vi "Center Insertion and IFFT.vi"(2 "Samples/Symbol":i32, 3 "Y(f) in":cdb[](array[numeric])) -> (0 "Freq Plot":dbl[](graph), 1 "Y(t) out":cdb[](array[numeric]))   [LabVIEW 2018]
uses:
  <vilib>/Analysis/NI_AALPro.lvlib
  <vilib>/Analysis/2dsp.llb/Inverse Complex FFT.vi
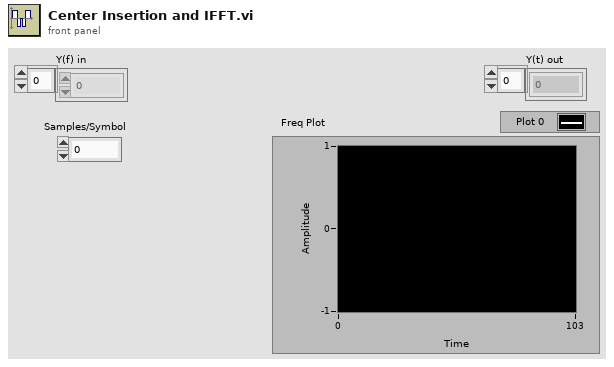
[diagram p1: front panel]
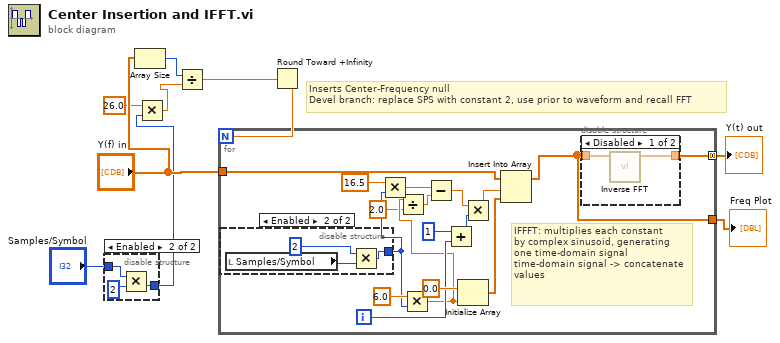
[diagram p0: block diagram]
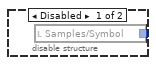
[diagram p3: hidden frame]
diagram:
  # "Inserts Center-Frequency null\nDevel branch: replace SPS with constant 2, use prior to waveform and recall FFT"
  n1 = disable-structure shown="Enabled" {
    disable-tunnel: [_ w13] -> w2
    disable-tunnel: "Samples/Symbol" -> [_ w11]
    frame Disabled {
    }
    frame Enabled {
      n2 = Multiply(x=w11, y=2) -> (x*y=w13:i32)
    }
  }
  n3 = Array Size(array="Y(f) in") -> (size(s)=w9:i32)
  n4 = Multiply(x=26.0, y=w2) -> (x*y=w3:dbl)
  n5 = Divide(x=w9, y=w3) -> (x/y=w10:dbl)
  n6 = Round Toward +Infinity(x=w10) -> (ceil(x): smallest int >= x=w8:dbl)
  n7 = for {
    N: w8 -> [_]
    tunnel: "Y(f) in" -> [w21]
    tunnel: [w23] -> w6 mode=concatenating
    tunnel: [w22] -> w5
    i -> [w27]
    # "IFFFT: multiplies each constant  \nby complex sinusoid, generating\none time-domain signal\ntime-domain signal -> concatenate values"
    n8 = disable-structure shown="Enabled" {
      disable-tunnel: [w31 w34] -> w19
      frame Disabled {
        n9 = local read "Samples/Symbol"() -> (w31:i32)
      }
      frame Enabled {
        n10 = local read "Samples/Symbol"() -> (w32:i32)
        n11 = Multiply(x=2 ("Samples/Symbol"), y=w32) -> (x*y=w34:i32)
      }
    }
    n12 = Multiply(x=16.5, y=w19) -> (x*y=w18:dbl)
    n13 = Multiply(x=6.0, y=w19) -> (x*y=w15:dbl)
    n14 = Divide(x=w15, y=2.0) -> (x/y=w16:dbl)
    n15 = Subtract(x=w18, y=w16) -> (x-y=w20:dbl)
    n16 = Add(x=1, y=w27) -> (x+y=w24:i32)
    n17 = Initialize Array(0.0 ("element"), w15) -> (w28:dbl[])
    n18 = Multiply(x=w20, y=w24) -> (x*y=w25:dbl)
    n19 = Insert Into Array(array=w21, index=w25, new element=w28) -> (w22:cdb[])
    n20 = disable-structure shown="Disabled" {
      disable-tunnel: [w36 w37] -> w23
      disable-tunnel: w22 -> [w35 w37]
      frame Disabled {
        n21 = call-poly <vilib>:"Inverse FFT.vi"("FFT {X}"=w35) -> ("X"=w36:cdb[])  [unwired: 9 in, 1 out]
      }
      frame Enabled {
      }
    }
  }
  "Y(t) out" <- w6
  "Freq Plot" <- w5
